vi "Main_10a.vi"() -> ()   [LabVIEW 2020]
panel:
  out "X":i32
  out "Value":i32[](array[numeric])
  in  "Example 2":string="addx 15\naddx -11\naddx 6\naddx -3\naddx 5\naddx -1\naddx -8\naddx 13\naddx 4\nnoop\naddx -1\naddx 5\naddx -1\naddx 5\naddx -1\naddx 5\naddx -1\naddx 5\naddx -1\naddx -35\naddx 1\naddx 24\naddx -19\naddx 1\naddx 16\naddx -11\nnoop\nnoop\naddx 21\naddx -15\nnoop\nnoop\naddx -3\naddx 9\naddx 1\naddx -3\naddx 8\naddx 1\naddx 5\nnoop\nnoop\nnoop\nnoop\nnoop\naddx -36\nnoop\naddx 1\naddx 7\nnoop\nnoop\nnoop\naddx 2\naddx 6\nnoop\nnoop\nnoop\nnoop\nnoop\naddx 1\nnoop\nnoop\naddx 7\naddx 1\nnoop\naddx -13\naddx 13\naddx 7\nnoop\naddx 1\naddx -33\nnoop\nnoop\nnoop\naddx 2\nnoop\nnoop\nnoop\naddx 8\nnoop\naddx -1\naddx 2\naddx 1\nnoop\naddx 17\naddx -9\naddx 1\naddx 1\naddx -3\naddx 11\nnoop\nnoop\naddx 1\nnoop\naddx 1\nnoop\nnoop\naddx -13\naddx -19\naddx 1\naddx 3\naddx 26\naddx -30\naddx 12\naddx -1\naddx 3\naddx 1\nnoop\nnoop\nnoop\naddx -9\naddx 18\naddx 1\naddx 2\nnoop\nnoop\naddx 9\nnoop\nnoop\nnoop\naddx -1\naddx 2\naddx -37\naddx 1\naddx 3\nnoop\naddx 15\naddx -21\naddx 22\naddx -6\naddx 1\nnoop\naddx 2\naddx 1\nnoop\naddx -10\nnoop\nnoop\naddx 20\naddx 1\naddx 2\naddx 2\naddx -6\naddx -11\nnoop\nnoop\nnoop"
  out "sum":i32
  in  "Puzzle":string="addx 1\naddx 5\nnoop\naddx -1\nnoop\naddx 3\naddx 29\naddx -1\naddx -21\naddx 5\nnoop\naddx -20\naddx 21\naddx 2\naddx 8\naddx -1\nnoop\nnoop\nnoop\nnoop\naddx 6\naddx -1\naddx -37\naddx 40\naddx -10\naddx -25\naddx 5\naddx 2\naddx 5\nnoop\nnoop\nnoop\naddx 21\naddx -20\naddx 2\nnoop\naddx 3\naddx 2\naddx -5\naddx 12\naddx 3\nnoop\naddx 2\naddx 3\naddx -2\naddx -37\naddx 1\naddx 5\naddx 3\naddx -2\naddx 2\naddx 29\naddx -22\naddx 13\nnoop\naddx -8\naddx -6\naddx 7\naddx 2\nnoop\naddx 7\naddx -2\naddx 5\naddx 2\naddx -26\naddx -11\nnoop\nnoop\naddx 6\naddx 1\naddx 1\nnoop\naddx 4\naddx 5\nnoop\nnoop\naddx -2\naddx 3\nnoop\naddx 2\naddx 5\naddx 2\naddx -22\naddx 27\naddx -1\naddx 1\naddx 5\naddx 2\nnoop\naddx -39\naddx 22\nnoop\naddx -15\naddx 3\naddx -2\naddx 2\naddx -2\naddx 9\naddx 3\nnoop\naddx 2\naddx 3\naddx -2\naddx 2\nnoop\nnoop\nnoop\naddx 5\naddx -17\naddx 24\naddx -7\naddx 8\naddx -36\naddx 2\naddx 3\naddx 33\naddx -32\naddx 4\naddx 1\nnoop\naddx 5\nnoop\nnoop\naddx 20\naddx -15\naddx 4\nnoop\naddx 1\nnoop\naddx 4\naddx 6\naddx -30\naddx 30\nnoop\nnoop\nnoop\nnoop\nnoop"
  in  "Example":string="noop\naddx 3\naddx -5"
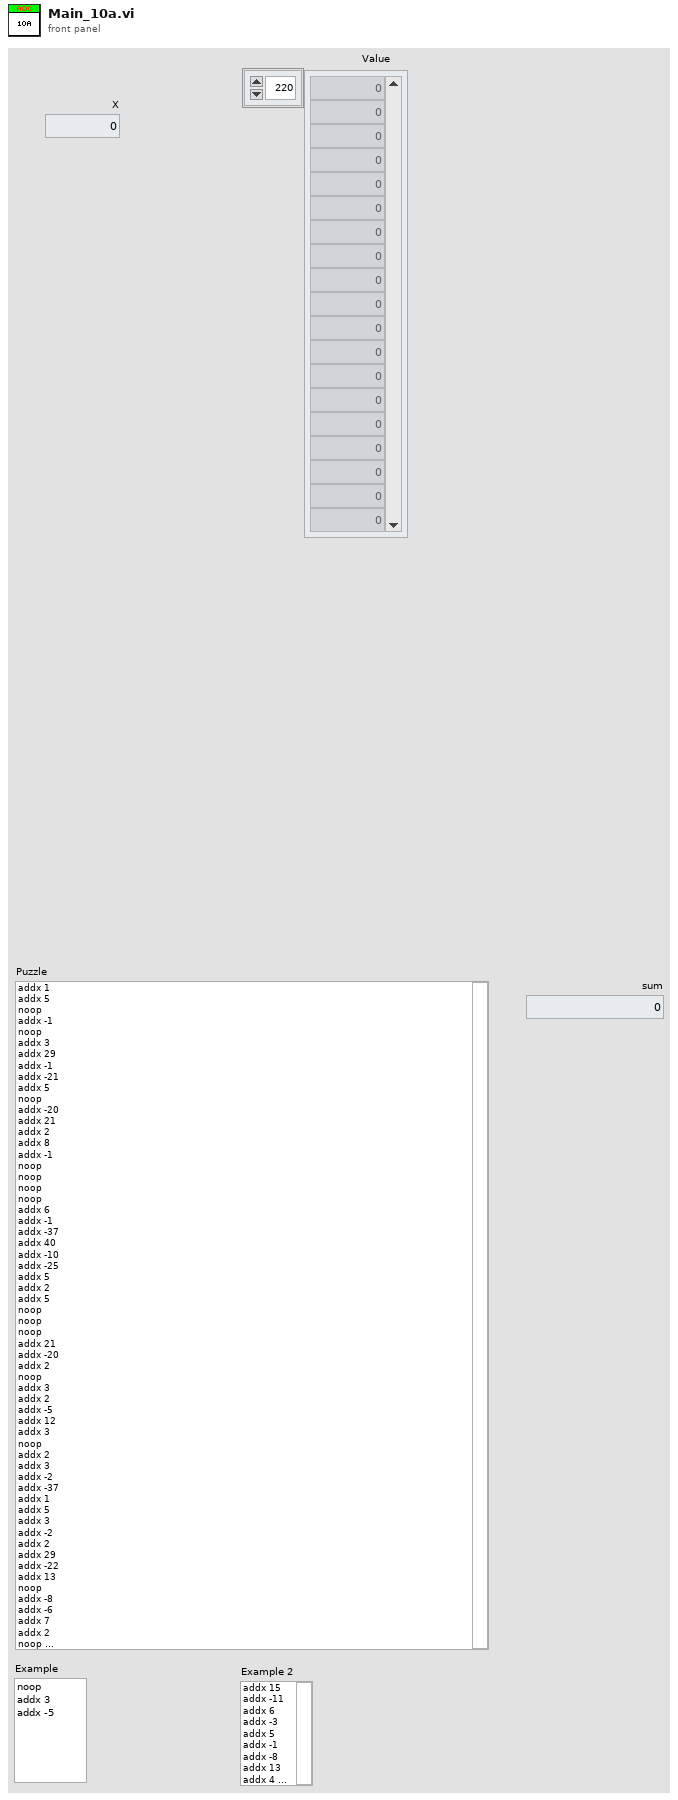
[diagram p1: front panel]
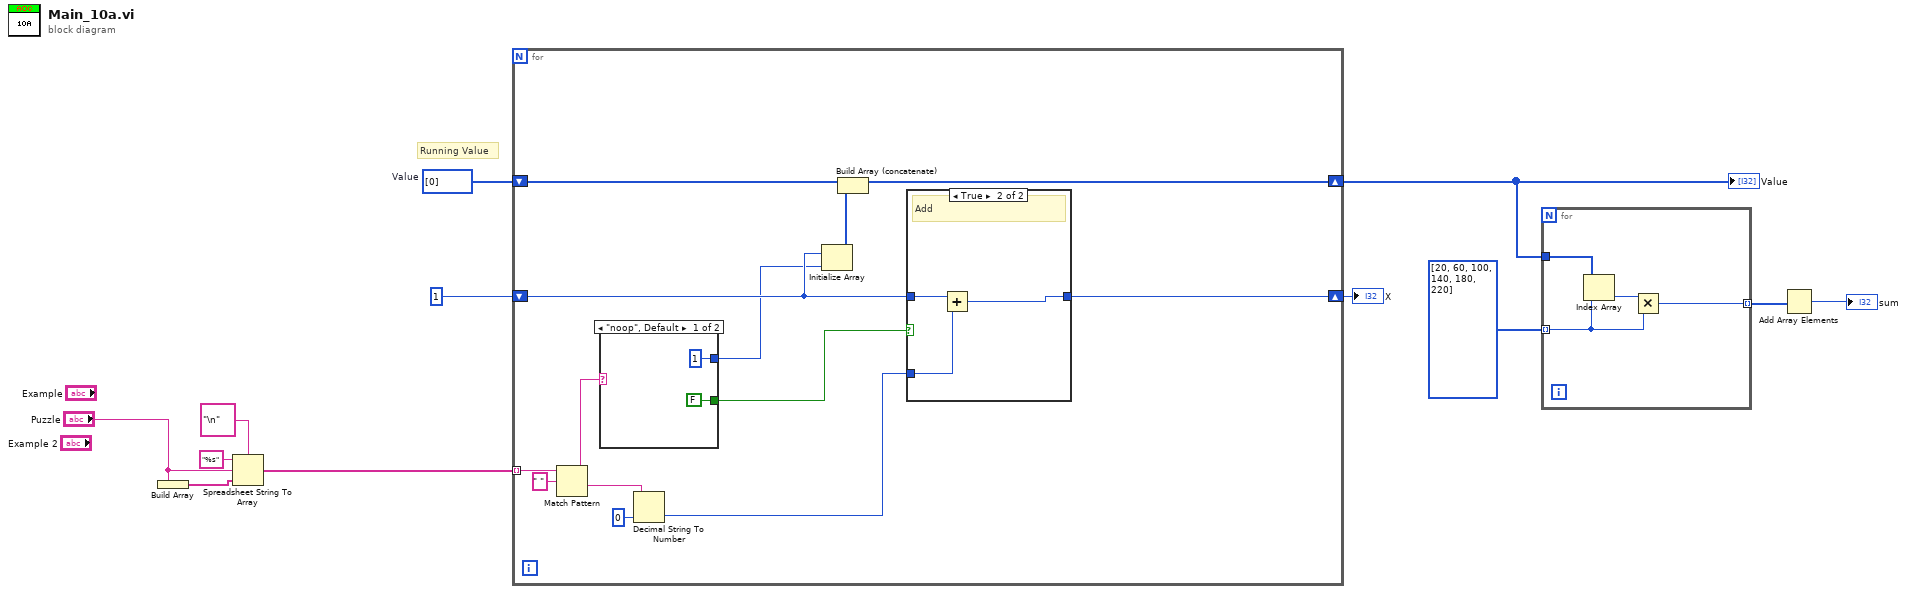
[diagram p0: block diagram]
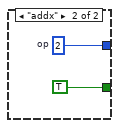
[diagram p2: hidden frame]
diagram:
  w9 = i32[] [0]  # Value
  # "Running Value"
  n1 = Build Array("Puzzle") -> (w7:string[])
  n2 = Spreadsheet String To Array(delimiter (Tab)="\n", format string="%s", spreadsheet string="Puzzle", array type (2D Dbl)=w7) -> (array=w8:string[])
  n3 = for {
    shift-right: [w21] -> w6
    shift-left: 1 -> [w23]
    shift-right: [w22] -> w4
    shift-left: w9 -> [w25]
    tunnel: w8 -> [w20] mode=indexing
    n4 = Match Pattern(string=w20, regular expression=" ") -> (before substring=w15:string, after substring=w19:string)  [unwired: 1 in, 2 out]
    n5 = case shown="\"noop\", Default" w15 {
      tunnel: [1 ("op") w29] -> w14
      tunnel: [FALSE TRUE] -> w13
      frame "noop", Default {
      }
      frame "addx" {
        w29 = 2  # op
      }
    }
    n6 = Decimal String To Number(string=w19, default (0L)=0 ("default (0 I32)")) -> (number=w16:i32)  [unwired: 1 in, 1 out]
    n7 = Initialize Array(w23, w14) -> (w24:i32[])
    n8 = Build Array (concatenate)(w25, w24) -> (w22:i32[])
    n9 = case shown="True" w13 {
      tunnel: w23 -> [w30 w33]
      tunnel: w16 -> [_ w32]
      tunnel: [w30 w31] -> w21
      frame False {
        # "noop"
      }
      frame True {
        # "Add"
        n10 = Add(x=w33, y=w32) -> (x+y=w31:i32)
      }
    }
  }
  "Value" <- w4
  "X" <- w6
  n11 = for {
    tunnel: i32[] [20, 60, 100, 140, 180, 220] ("Value") -> [w35] mode=indexing
    tunnel: w4 -> [w37]
    tunnel: [w34] -> w3 mode=indexing
    n12 = Index Array(array=w37, index=w35) -> (element=w36:i32)
    n13 = Multiply(x=w36, y=w35) -> (x*y=w34:i32)
  }
  n14 = Add Array Elements(numeric array=w3) -> (sum=→"sum":i32)
